vi "i2cbytearray2uSdistance.vi"(0 "Bytes read":u8[](array[numeric])) -> (1 "Distance - left":i32, 2 "Distance - right":i32)   [LabVIEW 2013]
uses:
  <vilib>/Utility/error.llb/whitespace.ctl
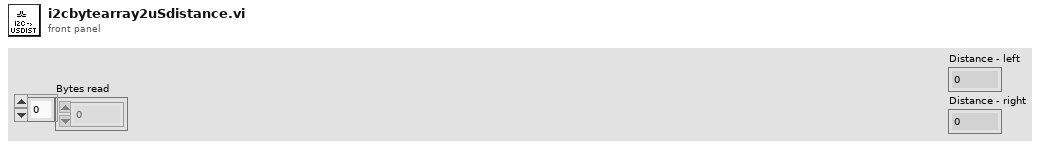
[diagram p1: front panel]
types:
  T1 = typedef "whitespace.ctl" = u16
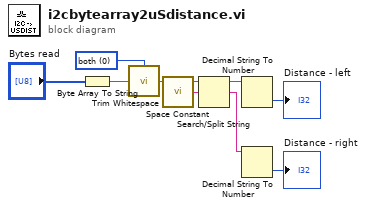
[diagram p0: block diagram]
diagram:
  w6 = T1 0 items=["both", "start of string", "end of string"] ("location (both)")
  n1 = Byte Array To String(unsigned byte array="Bytes read") -> (string=w7:string)
  n2 = call <vilib>:"Trim Whitespace.vi"("string"=w7, "location (both)"=w6) -> ("trimmed string"=w9:string)
  n3 = call <vilib>:"Space Constant.vi"() -> ("String"=w8:string)
  n4 = Search/Split String(string=w9, search string/char (-)=w8) -> (substring before match=w3:string, match + rest of string=w4:string)  [unwired: 1 in, 1 out]
  n5 = Decimal String To Number(string=w3) -> (number=→"Distance - left":i32)  [unwired: 2 in, 1 out]
  n6 = Decimal String To Number(string=w4) -> (number=→"Distance - right":i32)  [unwired: 2 in, 1 out]
